vi "closeFitsFile.vi"(8 "error in (no error)":errorcluster, 11 "Model in":refnum<class "Model.lvclass">) -> (0 "error out":errorcluster, 3 "Model out":refnum<class "Model.lvclass">)   [LabVIEW 2016, in "Model.lvclass"]
uses:
  Model.lvclass
  Model.lvclass/Model.ctl
  CFitsIO/CFitsIO.lvclass
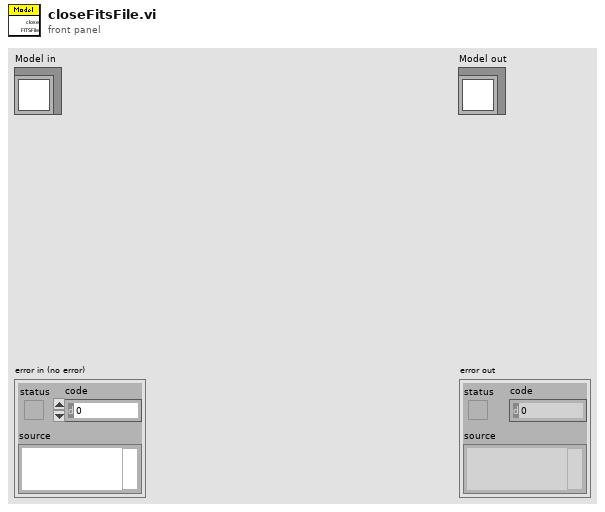
[diagram p1: front panel]
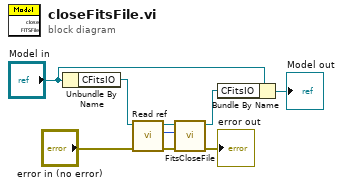
[diagram p0: block diagram]
diagram:
  n1 = Unbundle By Name("Model in") -> ("CFitsIO"=w9:refnum<class "CFitsIO.lvclass">)
  n2 = call-dynamic "Read ref .vi"("error in (no error)"="error in (no error)", "CFitsIO in"=w9) -> ("error out"=w5:errorcluster, "ref"=w6:u64, "CFitsIO out"=w7:refnum<class "CFitsIO.lvclass">)  [unwired: 7 in]
  n3 = call-dynamic "FitsCloseFile.vi"("error in (no error)"=w5, "ref in"=w6, "CFitsIO in"=w7) -> ("error out"=→"error out":errorcluster, "CFitsIO out"=w4:refnum<class "CFitsIO.lvclass">)  [unwired: 5 in, 2 out]
  n4 = Bundle By Name(cluster="Model in", "CFitsIO"=w4) -> (→"Model out":refnum<class "Model.lvclass">)
